vi "SENS_MULT_LAB.vi"(0 "VISA IN":refnum<visa-resource-name>, 1 "Display Label Text":string, 5 "error in":errorcluster, 7 "Channel":i32) -> (14 "VISA Out":refnum<visa-resource-name>, 19 "error out":errorcluster)   [LabVIEW 2018, in "PNA-X.lvlib"]
doc: "SENSe<cnum>:MULTiplexer:LABel <string> \n(Read-Write) Sets and returns the display label for the testset on the specified channel. The label \nappears in a status bar at the bottom of the PNA display when SENS:MULT:DISP is set to TRUE. \nParameters \n<cnum> Any existing channel number. If unspecified, value is set to 1. \n<string> Display label text. \nExamples SENS3:MULT:LAB 'High-power output' \nQuery Syntax SENSe<cnum>:MULTiplexer:LABel? \nReturn Type String \nDefault Not Applicable"
uses:
  PNA-X.lvlib
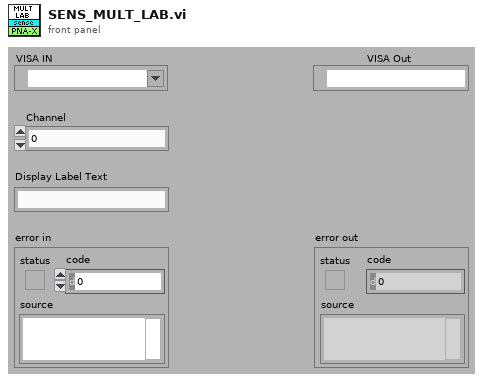
[diagram p1: front panel]
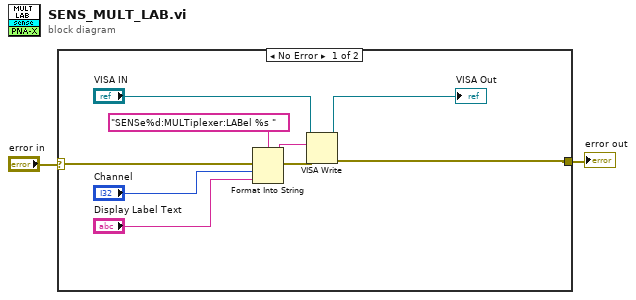
[diagram p0: block diagram]
diagram:
  n1 = case shown="No Error" "error in" {
    selector: "error in" -> [w11 w12]
    tunnel: [w6 w12] -> w1
    frame No Error {
      n2 = Format Into String(format string="SENSe%d:MULTiplexer:LABel %s " ("Cmdline"), error in=w11, "Channel", "Display Label Text") -> (resulting string=w9:string, error out=w10:errorcluster)  [unwired: 1 in]
      n3 = VISA Write(VISA resource name="VISA IN", write buffer=w9, error in (no error)=w10) -> (VISA resource name out=→"VISA Out":refnum<visa-resource-name>, error out=w6:errorcluster)  [unwired: 1 out]
    }
    frame Error {
    }
  }
  "error out" <- w1
